vi "HypervisorWrite.vi"(8 "ErrorIn":errorcluster, 10 "EventToLog":T1, 11 "QIn":refnum<queue>) -> (0 "ErrorOut":errorcluster, 3 "QOut":refnum<queue>)   [LabVIEW 2018]
doc: "This VI writes EventToLog to the Hypervisor log file.\n\nCopyright © 2019 Epimedia, Inc. All Rights Reserved.\n\nThe Epimedia Application Library is Copyright © 2009-2017 Epimedia, Inc. \nAll Rights Reserved. Used under license."
uses:
  Queue/HyperVisor.ctl
  <vilib>/Utility/sysdir.llb/System Directory Type.ctl
panel:
  # "Copyright © 2019 Epimedia, Inc. All Rights Reserved.\n\nThe Epimedia Application Library is Copyright © 2009-2017 Epimedia, Inc. \nAll Rights Reserved. Used under license."
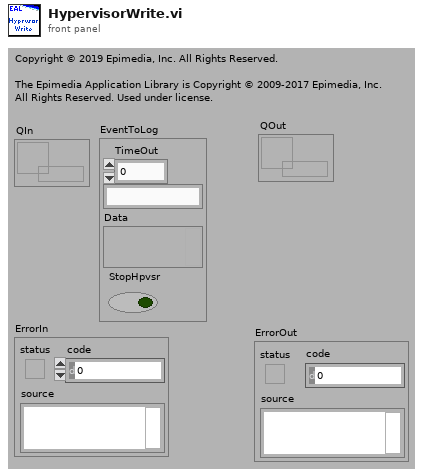
[diagram p1: front panel]
types:
  T1 = typedef "HyperVisor.ctl" = cluster{"TimeOut":dbl, string, "Data":variant, "StopHpvsr":bool}
  T2 = typedef "System Directory Type.ctl" = i32
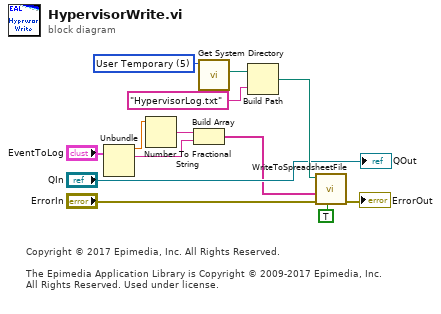
[diagram p0: block diagram]
diagram:
  w12 = T2 5 items=["User Home"=0, "User Desktop"=1, "User Documents"=2, "User Application Data"=3, "User Preferences"=4, "User Temporary"=5, "Public Documents"=6, "Public Application Data"=7, "Public Preferences"=8, "Public Cache"=13, "System Core Libraries"=9, "System Installed Libraries"=10, "Application Files"=11, "Boot Volume Root"=12] ("system directory type")
  # "Copyright © 2017 Epimedia, Inc. All Rights Reserved.\n\nThe Epimedia Application Library is Copyright © 2009-2017 Epimedia, Inc. \nAll Rights Reserved. Used under license."
  n1 = Unbundle("EventToLog") -> ("TimeOut"=w8:dbl, w7:string)  [unwired: 2 out]
  n2 = Number To Fractional String(number=w8) -> (F-format string=w6:string)  [unwired: 1 in, 2 out]
  n3 = Build Array(w6, w7) -> (w2:string[])
  n4 = call <vilib>:"Get System Directory.vi"("system directory type"=w12) -> ("system directory"=w11:path)  [unwired: 10 in]
  n5 = Build Path(base path=w11, name or relative path="HypervisorLog.txt") -> (appended path=w9:path)
  n6 = call "WriteToSpreadsheetFile.vi"("Append?(NewFile:F)"=TRUE ("append to file? (new file:F)"), "ErrorIn"="ErrorIn", "1D-Data"=w2, "FilePath(DialogIfEmpty)"=w9) -> ("ErrorOut"=→"ErrorOut":errorcluster)  [unwired: 4 in, 3 out]
  "QOut" <- "QIn"
